vi "MetersToPixels.vi"(1 "Arena Meters":dbl) -> (0 "Arena Pixels":dbl)   [LabVIEW 2015, in "Localization Mockup - DEPRECATED.lvlib"]
uses:
  Localization Mockup - DEPRECATED.lvlib
  Navigation2017.lvlib
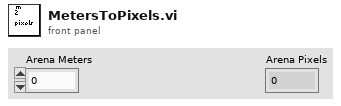
[diagram p1: front panel]
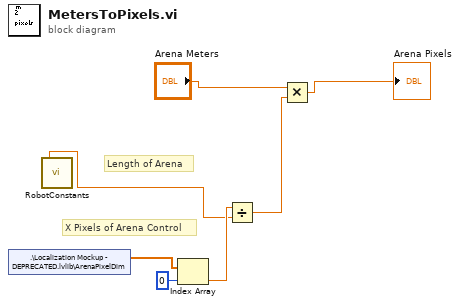
[diagram p0: block diagram]
diagram:
  # "X Pixels of Arena Control"
  # "Length of Arena"
  n1 = shared-variable ".\\Localization Mockup - DEPRECATED.lvlib\\ArenaPixelDim"() -> (w4:dbl[])  [unwired: 1 in, 1 out]
  n2 = call "RobotConstants.vi"() -> ("Arena Width (m)"=w1:dbl)  [unwired: 4 out]
  n3 = Index Array(array=w4, index=0) -> (element=w2:dbl)
  n4 = Divide(x=w2, y=w1) -> (x/y=w5:dbl)
  n5 = Multiply(x="Arena Meters", y=w5) -> (x*y=→"Arena Pixels":dbl)
